vi "ADL.vi"() -> ()   [LabVIEW 2017]
uses:
  Control/State.ctl
panel:
  in  "error in":errorcluster
  in  "Blender Path":string="\"C:\\Program Files\\Blender Foundation\\Blender 4.0\\blender.exe\""
  in  "Stop":bool
  in  "Start":bool
  in  "State":T1
  in  "ADL":u16(ring)=2 items=["None", "Book", "Pitcher", "Laptop", "Gear"]
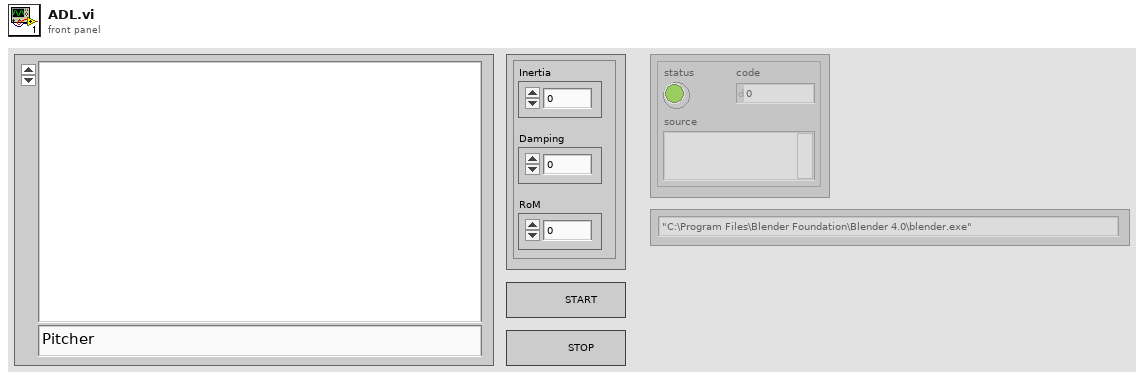
[diagram p1: front panel]
types:
  T1 = typedef "State.ctl" = cluster{"Inertia":dbl, "Damping":dbl, "RoM":dbl}
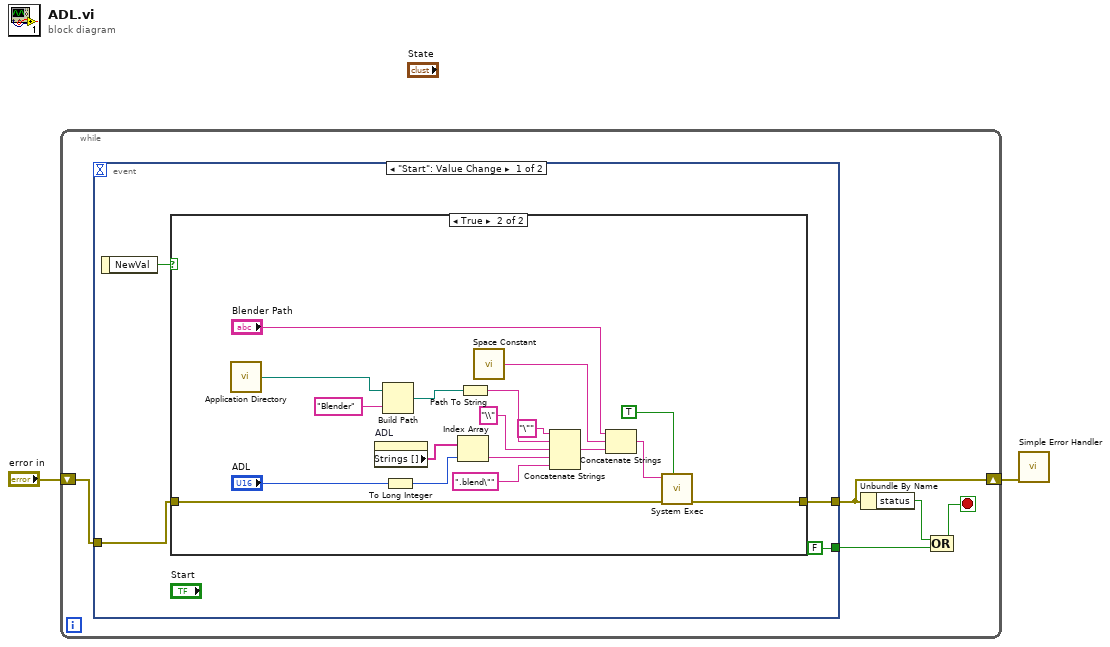
[diagram p0: block diagram]
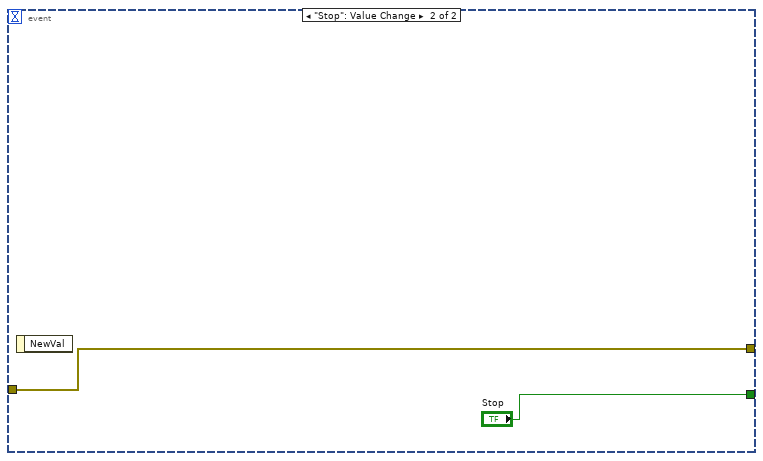
[diagram p3: hidden frame]
diagram:
  n1 = while {
    shift-right: [w6] -> w1
    shift-left: "error in" -> [w7]
    stop <- w3 stop-if-true
    n2 = event shown="[0] \"Start\": Value Change" {
      selector: _ -> [_ _]
      dyn-events: _ -> [_ _]
      timeout: _ -> [_ _]
      tunnel: [w10 w32] -> w6
      tunnel: w7 -> [w9 w32]
      tunnel: [FALSE ("Stop") "Stop"] -> w5
      event "Start": Value Change {
        n3 = event-data() -> ("NewVal"=w11:bool)  [unwired: 1 in]
        n4 = case shown="True" w11 {
          tunnel: [w12 w30] -> w10
          tunnel: w9 -> [w12 w29]
          frame False {
          }
          frame True {
            n5 = call <vilib>:"Application Directory.vi"() -> ("Application Directory"=w23:path)
            n6 = property on="ADL" class="Ring (strict)"() -> ("Strings []"=w28:string[])  [unwired: 2 in, 2 out]
            n7 = Build Path(base path=w23, name or relative path="Blender") -> (appended path=w21:path)
            n8 = To Long Integer(number="ADL") -> (32bit integer=w26:i32)
            n9 = Index Array(array=w28, index=w26) -> (element=w25:string)
            n10 = Path To String(path=w21) -> (string=w20:string)
            n11 = call <vilib>:"Space Constant.vi"() -> ("String"=w16:string)
            n12 = Concatenate Strings("\"" ("string"), w20, "\\" ("string"), w25, ".blend\"" ("string")) -> (w13:string)
            n13 = Concatenate Strings("Blender Path", w16, w13) -> (w15:string)
            n14 = call <vilib>:"System Exec.vi"("wait until completion? (T)"=TRUE, "error in (no error)"=w29, "command line"=w15) -> ("error out"=w30:errorcluster)  [unwired: 5 in, 3 out]
          }
        }
      }
      event "Stop": Value Change {
        n15 = event-data() -> ()  [unwired: 1 in, 1 out]
      }
    }
    n16 = Unbundle By Name(w6) -> ("status"=w4:bool)
    n17 = Compound Arithmetic op=OR(w4, w5) -> (w3:bool)
  }
  n18 = call <vilib>:"Simple Error Handler.vi"("error in (no error)"=w1) -> ()  [unwired: 4 in, 5 out]
